vi "CF_Write_Config.vi"(4 "error in (no error)":errorcluster, 7 "Config Refnum":T1) -> (0 "error out":errorcluster, 3 "refnum out":T1)   [LabVIEW 2015]
uses:
  <vilib>/Utility/config.llb/Config Data RefNum.ctl
  Systems/Cam_Focus/GSP_CF_Global.vi
  <vilib>/Utility/config.llb/Write Key (Double).vi
  <vilib>/Utility/config.llb/NI_LVConfig.lvlib
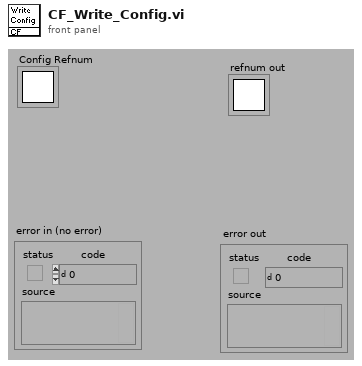
[diagram p1: front panel]
types:
  T1 = typedef "NI_LVConfig.lvlib/Config Data RefNum.ctl" = refnum<k1>
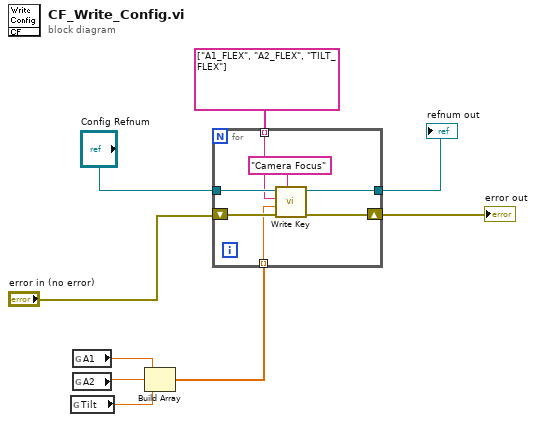
[diagram p0: block diagram]
diagram:
  n1 = global read "GSP_CF_Global.vi" "Tilt"() -> (w1:dbl)
  n2 = global read "GSP_CF_Global.vi" "A1"() -> (w3:dbl)
  n3 = global read "GSP_CF_Global.vi" "A2"() -> (w2:dbl)
  n4 = Build Array(w3, w2, w1) -> (w9:dbl[])
  n5 = for {
    tunnel: "Config Refnum" -> [w15]
    shift-right: [w13] -> w5
    shift-left: "error in (no error)" -> [w16]
    tunnel: [w12] -> w4
    tunnel: w9 -> [w10] mode=indexing
    tunnel: string[] ["A1_FLEX", "A2_FLEX", "TILT_FLEX"] -> [w11] mode=indexing
    n6 = call-poly <vilib>:"Write Key.vi"("section"="Camera Focus", "error in (no error)"=w16, "value"=w10, "key"=w11, "refnum"=w15) -> ("error out"=w13:errorcluster, "refnum out"=w12:T1)  [unwired: 4 in, 1 out]
  }
  "error out" <- w5
  "refnum out" <- w4
